vi "Test All.vi"() -> (2 "Failed Tests":i32[](array[numeric]), 3 "All Passed":bool)   [LabVIEW 2017]
uses:
  INI-Static-Variable-Support/LabVIEW-Config/Write Key (Boolean).vi
  INI-Static-Variable-Support/LabVIEW-Config/Read Key (Boolean).vi
  INI-Static-Variable-Support/LabVIEW-Config/Write Key (I32).vi
  INI-Static-Variable-Support/LabVIEW-Config/Read Key (I32).vi
  INI-Static-Variable-Support/LabVIEW-Config/Write Key (U32).vi
  INI-Static-Variable-Support/LabVIEW-Config/Read Key (U32).vi
  INI-Static-Variable-Support/LabVIEW-Config/Write Key (DBL).vi
  INI-Static-Variable-Support/LabVIEW-Config/Read Key (DBL).vi
  INI-Static-Variable-Support/LabVIEW-Config/Write Key (String).vi
  INI-Static-Variable-Support/LabVIEW-Config/Read Key (String).vi
  INI-Static-Variable-Support/LabVIEW-Config/LabVIEW-Config.lvlib
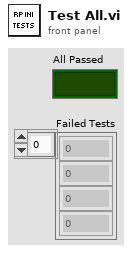
[diagram p1: front panel]
types:
  T1 = typedef "LabVIEW-Config.lvlib/Config.ctl" = cluster{"Path":path, "Lines":string[], "Tokens":enum8{"comment", "section", "key"}[], "Modified?":bool}
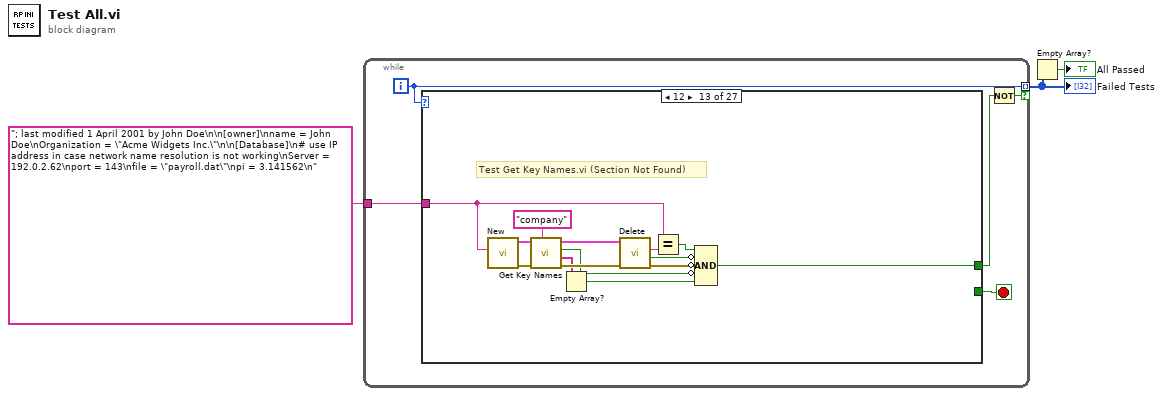
[diagram p0: block diagram]
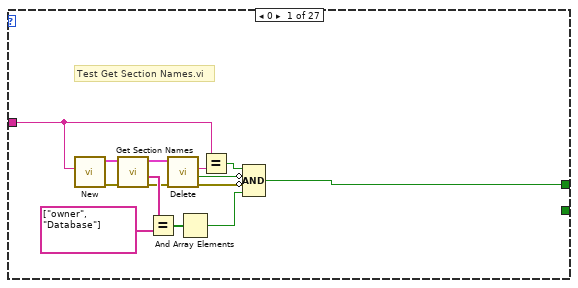
[diagram p2: hidden frame]
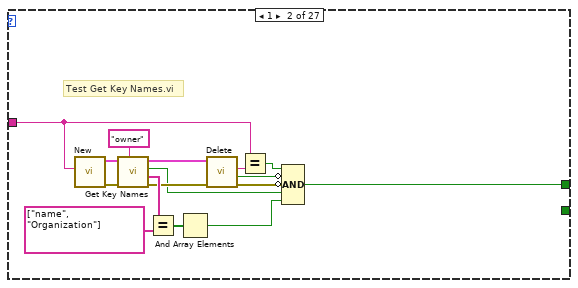
[diagram p3: hidden frame]
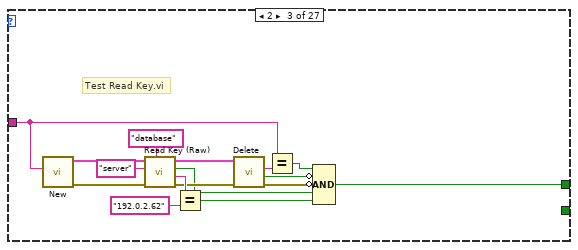
[diagram p4: hidden frame]
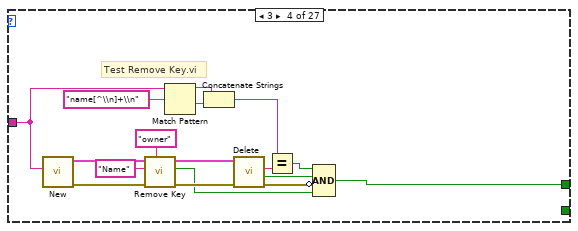
[diagram p5: hidden frame]
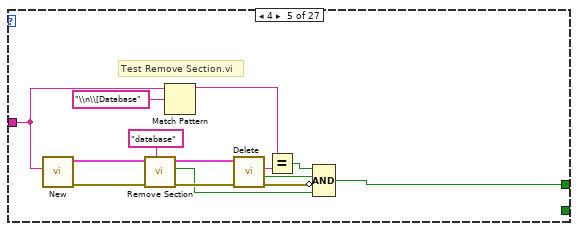
[diagram p6: hidden frame]
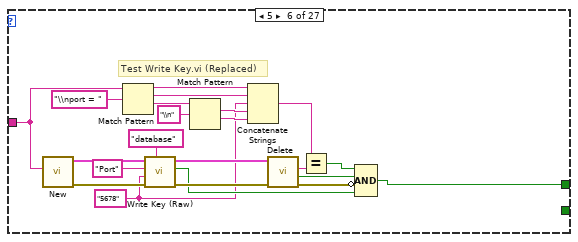
[diagram p7: hidden frame]
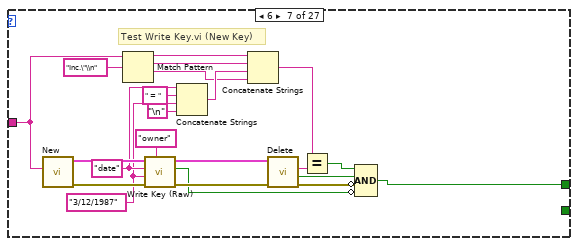
[diagram p8: hidden frame]
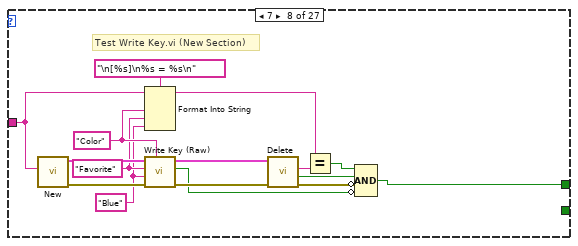
[diagram p9: hidden frame]
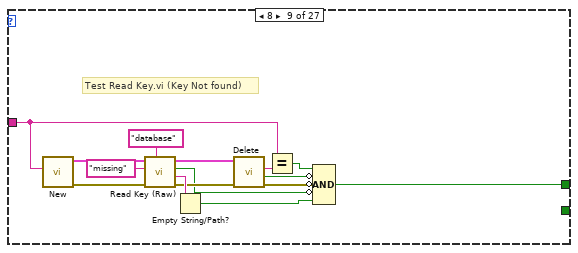
[diagram p10: hidden frame]
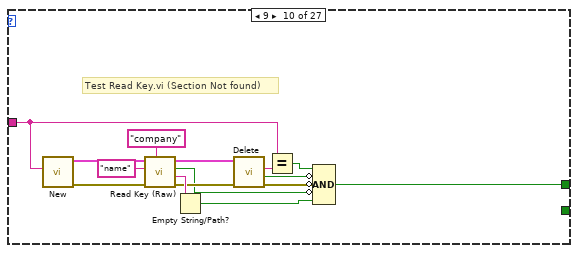
[diagram p11: hidden frame]
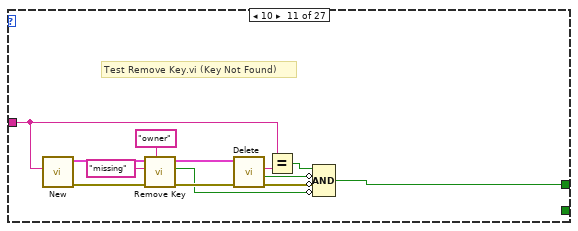
[diagram p12: hidden frame]
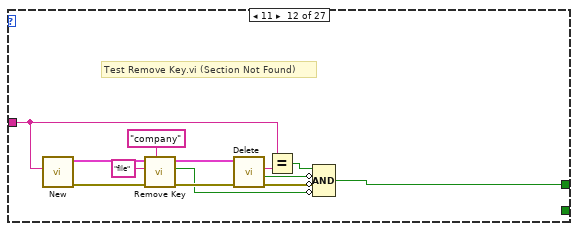
[diagram p13: hidden frame]
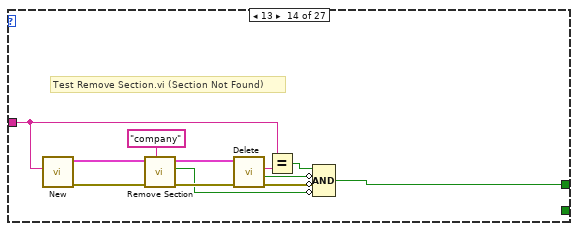
[diagram p14: hidden frame]
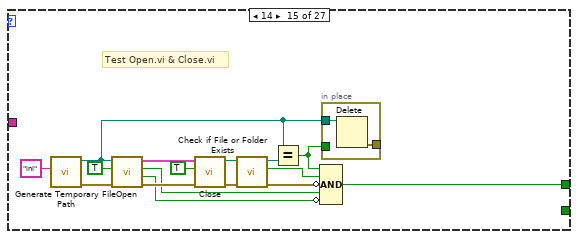
[diagram p15: hidden frame]
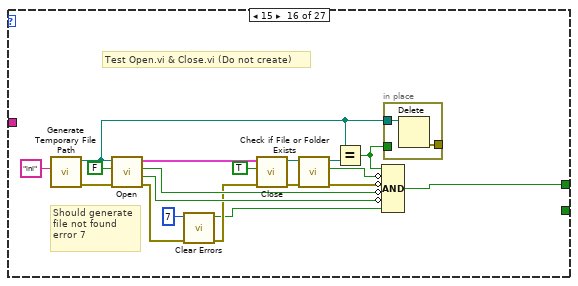
[diagram p16: hidden frame]
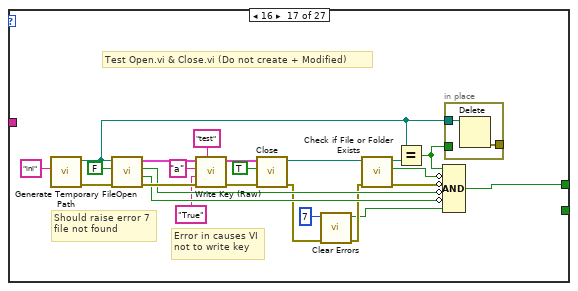
[diagram p17: hidden frame]
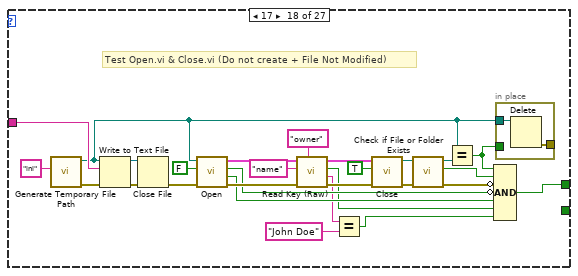
[diagram p18: hidden frame]
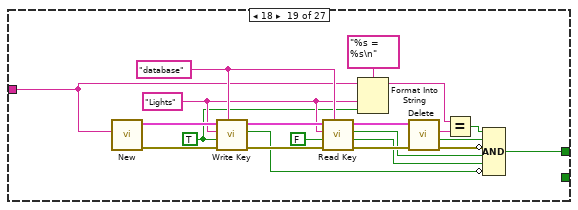
[diagram p19: hidden frame]
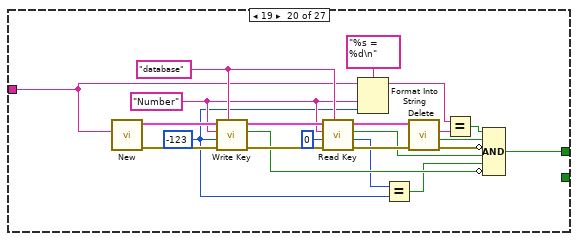
[diagram p20: hidden frame]
diagram:
  n1 = while {
    tunnel: "; last modified 1 April 2001 by John Doe\n\n[owner]\nname = John Doe\nOrganization = \"Acme Widgets Inc.\"\n\n[Database]\n# use IP address in case network name resolution is not working\nServer = 192.0.2.62\nport = 143\nfile = \"payroll.dat\"\npi = 3.141562\n" ("String") -> [w6]
    tunnel: [w7] -> w2 mode=indexing if=w4
    i -> [w7]
    stop <- w8 stop-if-true
    n2 = case shown="12" w7 {
      tunnel: [_ _ _ _ _ _ _ _ _ _ _ _ _ _ _ _ _ _ _ _ _ _ _ _ _ _ TRUE] -> w8
      tunnel: w6 -> [w14 w30 w48 w56 w74 w96 w118 w131 w154 w169 w176 w189 w210 w216 _ _ _ w296 w333 w355 w377 w403 w427 w451 w475 w499 _]
      tunnel: [w10 w24 w43 w62 w76 w98 w120 w137 w149 w164 w179 w192 w205 w218 w234 w255 w283 w313 w325 w348 w370 w396 w420 w444 w468 w492 TRUE] -> w5
      frame 0 {
        # "Test Get Section Names.vi"
        n3 = call "New.vi"("Text"=w14) -> ("error out"=w19:errorcluster, "Config"=w18:T1)  [unwired: 9 in]
        n4 = call "Get Section Names.vi"("error in (no error)"=w19, "Config in"=w18) -> ("error out"=w17:errorcluster, "Section Names"=w22:string[], "Config out"=w16:T1)  [unwired: 7 in]
        n5 = Equal?(x=w22, y=string[] ["owner", "Database"]) -> (x = y?=w20:bool[])
        n6 = call "Delete.vi"("error in (no error)"=w17, "Config"=w16) -> ("error out"=w13:errorcluster, "Modified?"=w9:bool, "Text"=w15:string)  [unwired: 6 in, 1 out]
        n7 = And Array Elements(Boolean array=w20) -> (logical AND=w11:bool)
        n8 = Equal?(x=w14, y=w15) -> (x = y?=w12:bool)
        n9 = Compound Arithmetic op=AND(w12, invert w9, invert w13, w11) -> (w10:bool)
      }
      frame 1 {
        # "Test Get Key Names.vi"
        n10 = call "New.vi"("Text"=w30) -> ("error out"=w35:errorcluster, "Config"=w34:T1)  [unwired: 9 in]
        n11 = call "Get Key Names.vi"("Section Name"="owner", "error in (no error)"=w35, "Config in"=w34) -> ("error out"=w33:errorcluster, "Key Names"=w38:string[], "Section Found?"=w25:bool, "Config out"=w32:T1)  [unwired: 5 in]
        n12 = Equal?(x=w38, y=string[] ["name", "Organization"]) -> (x = y?=w36:bool[])
        n13 = And Array Elements(Boolean array=w36) -> (logical AND=w26:bool)
        n14 = call "Delete.vi"("error in (no error)"=w33, "Config"=w32) -> ("error out"=w28:errorcluster, "Modified?"=w23:bool, "Text"=w31:string)  [unwired: 6 in, 1 out]
        n15 = Equal?(x=w30, y=w31) -> (x = y?=w27:bool)
        n16 = Compound Arithmetic op=AND(w27, invert w23, invert w28, w25, w26) -> (w24:bool)
      }
      frame 2 {
        # "Test Read Key.vi"
        n17 = call "New.vi"("Text"=w48) -> ("error out"=w53:errorcluster, "Config"=w52:T1)  [unwired: 9 in]
        n18 = call "Read Key (Raw).vi"("Section Name"="database", "error in (no error)"=w53, "Key Name"="server", "Config in"=w52) -> ("error out"=w51:errorcluster, "Content"=w54:string, "Key Found?"=w44:bool, "Config out"=w50:T1)  [unwired: 4 in]
        n19 = Equal?(x=w54, y="192.0.2.62") -> (x = y?=w40:bool)
        n20 = call "Delete.vi"("error in (no error)"=w51, "Config"=w50) -> ("error out"=w46:errorcluster, "Modified?"=w39:bool, "Text"=w49:string)  [unwired: 6 in, 1 out]
        n21 = Equal?(x=w48, y=w49) -> (x = y?=w45:bool)
        n22 = Compound Arithmetic op=AND(w45, invert w39, invert w46, w44, w40) -> (w43:bool)
      }
      frame 3 {
        # "Test Remove Key.vi"
        n23 = call "New.vi"("Text"=w56) -> ("error out"=w71:errorcluster, "Config"=w70:T1)  [unwired: 9 in]
        n24 = call "Remove Key.vi"("Section Name"="owner", "error in (no error)"=w71, "Key Name"="Name", "Config in"=w70) -> ("error out"=w69:errorcluster, "Key Found?"=w63:bool, "Config out"=w68:T1)  [unwired: 5 in]
        n25 = Match Pattern(string=w56, regular expression="name[^\\n]+\\n") -> (before substring=w59:string, after substring=w58:string)  [unwired: 1 in, 2 out]
        n26 = Concatenate Strings(w59, w58) -> (w57:string)
        n27 = call "Delete.vi"("error in (no error)"=w69, "Config"=w68) -> ("error out"=w65:errorcluster, "Modified?"=w55:bool, "Text"=w67:string)  [unwired: 6 in, 1 out]
        n28 = Equal?(x=w57, y=w67) -> (x = y?=w64:bool)
        n29 = Compound Arithmetic op=AND(w64, w55, invert w65, w63) -> (w62:bool)
      }
      frame 4 {
        # "Test Remove Section.vi"
        n30 = call "New.vi"("Text"=w74) -> ("error out"=w85:errorcluster, "Config"=w84:T1)  [unwired: 9 in]
        n31 = call "Remove Section.vi"("Section Name"="database", "error in (no error)"=w85, "Config in"=w84) -> ("error out"=w83:errorcluster, "Section Found?"=w77:bool, "Config out"=w82:T1)  [unwired: 6 in]
        n32 = Match Pattern(string=w74, regular expression="\\n\\[Database") -> (before substring=w73:string)  [unwired: 1 in, 3 out]
        n33 = call "Delete.vi"("error in (no error)"=w83, "Config"=w82) -> ("error out"=w79:errorcluster, "Modified?"=w72:bool, "Text"=w81:string)  [unwired: 6 in, 1 out]
        n34 = Equal?(x=w73, y=w81) -> (x = y?=w78:bool)
        n35 = Compound Arithmetic op=AND(w78, w72, invert w79, w77) -> (w76:bool)
      }
      frame 5 {
        w88 = "5678" ("Content")
        # "Test Write Key.vi (Replaced)"
        n36 = call "New.vi"("Text"=w96) -> ("error out"=w107:errorcluster, "Config"=w106:T1)  [unwired: 9 in]
        n37 = Match Pattern(string=w96, regular expression="\\nport = ") -> (before substring=w90:string, match substring=w87:string, after substring=w94:string)  [unwired: 1 in, 1 out]
        n38 = call "Write Key (Raw).vi"("Section Name"="database", "error in (no error)"=w107, "Content"=w88, "Key Name"="Port", "Config in"=w106) -> ("error out"=w105:errorcluster, "Key Replaced?"=w99:bool, "Config out"=w104:T1)  [unwired: 4 in]
        n39 = Match Pattern(string=w94, regular expression="\\n") -> (match substring=w92:string, after substring=w91:string)  [unwired: 1 in, 2 out]
        n40 = Concatenate Strings(w90, w87, w88, w92, w91) -> (w89:string)
        n41 = call "Delete.vi"("error in (no error)"=w105, "Config"=w104) -> ("error out"=w101:errorcluster, "Modified?"=w86:bool, "Text"=w103:string)  [unwired: 6 in, 1 out]
        n42 = Equal?(x=w89, y=w103) -> (x = y?=w100:bool)
        n43 = Compound Arithmetic op=AND(w100, w86, invert w101, w99) -> (w98:bool)
      }
      frame 6 {
        w112 = "3/12/1987" ("Content")
        w114 = "date" ("Key Name")
        # "Test Write Key.vi (New Key)"
        n44 = call "New.vi"("Text"=w118) -> ("error out"=w129:errorcluster, "Config"=w128:T1)  [unwired: 9 in]
        n45 = Match Pattern(string=w118, regular expression="Inc.\"\\n") -> (before substring=w117:string, match substring=w115:string, after substring=w109:string)  [unwired: 1 in, 1 out]
        n46 = call "Write Key (Raw).vi"("Section Name"="owner", "error in (no error)"=w129, "Content"=w112, "Key Name"=w114, "Config in"=w128) -> ("error out"=w127:errorcluster, "Key Replaced?"=w121:bool, "Config out"=w126:T1)  [unwired: 4 in]
        n47 = Concatenate Strings(w114, " = " ("string"), w112, "\n" ("Line Feed Constant")) -> (w111:string)
        n48 = Concatenate Strings(w117, w115, w111, w109) -> (w116:string)
        n49 = call "Delete.vi"("error in (no error)"=w127, "Config"=w126) -> ("error out"=w123:errorcluster, "Modified?"=w108:bool, "Text"=w125:string)  [unwired: 6 in, 1 out]
        n50 = Equal?(x=w116, y=w125) -> (x = y?=w122:bool)
        n51 = Compound Arithmetic op=AND(w122, w108, invert w123, invert w121) -> (w120:bool)
      }
      frame 7 {
        w133 = "Blue" ("Content")
        w134 = "Favorite" ("Key Name")
        w135 = "Color" ("Section Name")
        # "Test Write Key.vi (New Section)"
        n52 = call "New.vi"("Text"=w131) -> ("error out"=w145:errorcluster, "Config"=w144:T1)  [unwired: 9 in]
        n53 = Format Into String(format string="\n[%s]\n%s = %s\n", initial string=w131, w135, w134, w133) -> (resulting string=w130:string)  [unwired: 1 in, 1 out]
        n54 = call "Write Key (Raw).vi"("Section Name"=w135, "error in (no error)"=w145, "Content"=w133, "Key Name"=w134, "Config in"=w144) -> ("error out"=w143:errorcluster, "Key Replaced?"=w138:bool, "Config out"=w142:T1)  [unwired: 4 in]
        n55 = call "Delete.vi"("error in (no error)"=w143, "Config"=w142) -> ("error out"=w140:errorcluster, "Modified?"=w136:bool, "Text"=w141:string)  [unwired: 6 in, 1 out]
        n56 = Equal?(x=w130, y=w141) -> (x = y?=w139:bool)
        n57 = Compound Arithmetic op=AND(w139, w136, invert w140, invert w138) -> (w137:bool)
      }
      frame 8 {
        # "Test Read Key.vi (Key Not found)"
        n58 = call "New.vi"("Text"=w154) -> ("error out"=w159:errorcluster, "Config"=w158:T1)  [unwired: 9 in]
        n59 = call "Read Key (Raw).vi"("Section Name"="database", "error in (no error)"=w159, "Key Name"="missing", "Config in"=w158) -> ("error out"=w157:errorcluster, "Content"=w160:string, "Key Found?"=w150:bool, "Config out"=w156:T1)  [unwired: 4 in]
        n60 = Empty String/Path?(string/path=w160) -> (empty?=w147:bool)
        n61 = call "Delete.vi"("error in (no error)"=w157, "Config"=w156) -> ("error out"=w152:errorcluster, "Modified?"=w146:bool, "Text"=w155:string)  [unwired: 6 in, 1 out]
        n62 = Equal?(x=w154, y=w155) -> (x = y?=w151:bool)
        n63 = Compound Arithmetic op=AND(w151, invert w146, invert w152, invert w150, w147) -> (w149:bool)
      }
      frame 9 {
        # "Test Read Key.vi (Section Not found)"
        n64 = call "New.vi"("Text"=w169) -> ("error out"=w174:errorcluster, "Config"=w173:T1)  [unwired: 9 in]
        n65 = call "Read Key (Raw).vi"("Section Name"="company", "error in (no error)"=w174, "Key Name"="name", "Config in"=w173) -> ("error out"=w172:errorcluster, "Content"=w175:string, "Key Found?"=w165:bool, "Config out"=w171:T1)  [unwired: 4 in]
        n66 = Empty String/Path?(string/path=w175) -> (empty?=w162:bool)
        n67 = call "Delete.vi"("error in (no error)"=w172, "Config"=w171) -> ("error out"=w167:errorcluster, "Modified?"=w161:bool, "Text"=w170:string)  [unwired: 6 in, 1 out]
        n68 = Equal?(x=w169, y=w170) -> (x = y?=w166:bool)
        n69 = Compound Arithmetic op=AND(w166, invert w161, invert w167, invert w165, w162) -> (w164:bool)
      }
      frame 10 {
        # "Test Remove Key.vi (Key Not Found)"
        n70 = call "New.vi"("Text"=w176) -> ("error out"=w188:errorcluster, "Config"=w187:T1)  [unwired: 9 in]
        n71 = call "Remove Key.vi"("Section Name"="owner", "error in (no error)"=w188, "Key Name"="missing", "Config in"=w187) -> ("error out"=w186:errorcluster, "Key Found?"=w180:bool, "Config out"=w185:T1)  [unwired: 5 in]
        n72 = call "Delete.vi"("error in (no error)"=w186, "Config"=w185) -> ("error out"=w182:errorcluster, "Modified?"=w177:bool, "Text"=w184:string)  [unwired: 6 in, 1 out]
        n73 = Equal?(x=w176, y=w184) -> (x = y?=w181:bool)
        n74 = Compound Arithmetic op=AND(w181, invert w177, invert w182, invert w180) -> (w179:bool)
      }
      frame 11 {
        # "Test Remove Key.vi (Section Not Found)"
        n75 = call "New.vi"("Text"=w189) -> ("error out"=w201:errorcluster, "Config"=w200:T1)  [unwired: 9 in]
        n76 = call "Remove Key.vi"("Section Name"="company", "error in (no error)"=w201, "Key Name"="file", "Config in"=w200) -> ("error out"=w199:errorcluster, "Key Found?"=w193:bool, "Config out"=w198:T1)  [unwired: 5 in]
        n77 = call "Delete.vi"("error in (no error)"=w199, "Config"=w198) -> ("error out"=w195:errorcluster, "Modified?"=w190:bool, "Text"=w197:string)  [unwired: 6 in, 1 out]
        n78 = Equal?(x=w189, y=w197) -> (x = y?=w194:bool)
        n79 = Compound Arithmetic op=AND(w194, invert w190, invert w195, invert w193) -> (w192:bool)
      }
      frame 12 {
        # "Test Get Key Names.vi (Section Not Found)"
        n80 = call "New.vi"("Text"=w210) -> ("error out"=w215:errorcluster, "Config"=w214:T1)  [unwired: 9 in]
        n81 = call "Get Key Names.vi"("Section Name"="company", "error in (no error)"=w215, "Config in"=w214) -> ("error out"=w213:errorcluster, "Key Names"=w203:string[], "Section Found?"=w206:bool, "Config out"=w212:T1)  [unwired: 5 in]
        n82 = Empty Array?(array=w203) -> (empty?=w202:bool)
        n83 = call "Delete.vi"("error in (no error)"=w213, "Config"=w212) -> ("error out"=w208:errorcluster, "Modified?"=w204:bool, "Text"=w211:string)  [unwired: 6 in, 1 out]
        n84 = Equal?(x=w210, y=w211) -> (x = y?=w207:bool)
        n85 = Compound Arithmetic op=AND(w207, invert w204, invert w208, invert w206, w202) -> (w205:bool)
      }
      frame 13 {
        # "Test Remove Section.vi (Section Not Found)"
        n86 = call "New.vi"("Text"=w216) -> ("error out"=w227:errorcluster, "Config"=w226:T1)  [unwired: 9 in]
        n87 = call "Remove Section.vi"("Section Name"="company", "error in (no error)"=w227, "Config in"=w226) -> ("error out"=w225:errorcluster, "Section Found?"=w219:bool, "Config out"=w224:T1)  [unwired: 6 in]
        n88 = call "Delete.vi"("error in (no error)"=w225, "Config"=w224) -> ("error out"=w221:errorcluster, "Modified?"=w217:bool, "Text"=w223:string)  [unwired: 6 in, 1 out]
        n89 = Equal?(x=w216, y=w223) -> (x = y?=w220:bool)
        n90 = Compound Arithmetic op=AND(w220, invert w217, invert w221, invert w219) -> (w218:bool)
      }
      frame 14 {
        # "Test Open.vi & Close.vi"
        n91 = call <vilib>:"Generate Temporary File Path.vi"("Temporary File Extension (tmp)"="ini") -> ("error out"=w240:errorcluster, "Unique Temporary File Path"=w233:path)  [unwired: 9 in]
        n92 = call "Open.vi"("error in (no error)"=w240, "Create if not exists? (T)"=TRUE, "Path"=w233) -> ("error out"=w243:errorcluster, "File Exists?"=w235:bool, "File Created?"=w236:bool, "Config"=w242:T1)  [unwired: 5 in]
        n93 = call "Close.vi"("error in (no error)"=w243, "Write if modified? (T)"=TRUE, "Config"=w242) -> ("error out"=w237:errorcluster, "Path"=w230:path)  [unwired: 7 in]
        n94 = call <vilib>:"Check if File or Folder Exists.vi"("error in (no error)"=w237, "path"=w230) -> ("error out"=w231:errorcluster, "file or folder exists?"=w228:bool, "dup path"=w229:path)  [unwired: 7 in]
        n95 = Equal?(x=w233, y=w229) -> (x = y?=w232:bool)
        n96 = Compound Arithmetic op=AND(w232, w228, invert w231, w236, invert w235) -> (w234:bool)
        n97 = in-place {
          in-place-border: w233 -> [w245]
          in-place-border: w232 -> [_]
          in-place-border: [w244] -> _
          n98 = Delete(path (use dialog)=w245) -> (error out=w244:errorcluster)  [unwired: 4 in, 2 out]
        }
      }
      frame 15 {
        # "Should generate\nfile not found\nerror 7"
        # "Test Open.vi & Close.vi (Do not create)"
        n99 = call <vilib>:"Generate Temporary File Path.vi"("Temporary File Extension (tmp)"="ini") -> ("error out"=w261:errorcluster, "Unique Temporary File Path"=w254:path)  [unwired: 9 in]
        n100 = call "Open.vi"("error in (no error)"=w261, "Create if not exists? (T)"=FALSE, "Path"=w254) -> ("error out"=w264:errorcluster, "File Exists?"=w256:bool, "File Created?"=w257:bool, "Config"=w263:T1)  [unwired: 5 in]
        n101 = call <vilib>:"Clear Errors.vi"("error in (no error)"=w264, "specific error code to clear (0: all)"=7) -> ("error out"=w248:errorcluster, "specific error cleared?"=w246:bool)  [unwired: 4 in]
        n102 = call "Close.vi"("error in (no error)"=w248, "Write if modified? (T)"=TRUE, "Config"=w263) -> ("error out"=w258:errorcluster, "Path"=w251:path)  [unwired: 7 in]
        n103 = call <vilib>:"Check if File or Folder Exists.vi"("error in (no error)"=w258, "path"=w251) -> ("error out"=w252:errorcluster, "file or folder exists?"=w249:bool, "dup path"=w250:path)  [unwired: 7 in]
        n104 = Equal?(x=w254, y=w250) -> (x = y?=w253:bool)
        n105 = Compound Arithmetic op=AND(w253, invert w249, invert w252, invert w257, invert w256, w246) -> (w255:bool)
        n106 = in-place {
          in-place-border: w254 -> [w266]
          in-place-border: w253 -> [_]
          in-place-border: [w265] -> _
          n107 = Delete(path (use dialog)=w266) -> (error out=w265:errorcluster)  [unwired: 4 in, 2 out]
        }
      }
      frame 16 {
        # "Error in causes VI\nnot to write key"
        # "Should raise error 7\nfile not found"
        # "Test Open.vi & Close.vi (Do not create + Modified)"
        n108 = call <vilib>:"Generate Temporary File Path.vi"("Temporary File Extension (tmp)"="ini") -> ("error out"=w288:errorcluster, "Unique Temporary File Path"=w282:path)  [unwired: 9 in]
        n109 = call "Open.vi"("error in (no error)"=w288, "Create if not exists? (T)"=FALSE, "Path"=w282) -> ("error out"=w290:errorcluster, "File Exists?"=w284:bool, "File Created?"=w285:bool, "Config"=w275:T1)  [unwired: 5 in]
        n110 = call "Write Key (Raw).vi"("Section Name"="test", "error in (no error)"=w290, "Content"="True", "Key Name"="a", "Config in"=w275) -> ("error out"=w276:errorcluster, "Config out"=w274:T1)  [unwired: 4 in, 1 out]
        n111 = call "Close.vi"("error in (no error)"=w276, "Write if modified? (T)"=TRUE, "Config"=w274) -> ("error out"=w269:errorcluster, "Path"=w279:path)  [unwired: 7 in]
        n112 = call <vilib>:"Clear Errors.vi"("error in (no error)"=w269, "specific error code to clear (0: all)"=7) -> ("error out"=w268:errorcluster, "specific error cleared?"=w267:bool)  [unwired: 4 in]
        n113 = call <vilib>:"Check if File or Folder Exists.vi"("error in (no error)"=w268, "path"=w279) -> ("error out"=w280:errorcluster, "file or folder exists?"=w277:bool, "dup path"=w278:path)  [unwired: 7 in]
        n114 = Equal?(x=w282, y=w278) -> (x = y?=w281:bool)
        n115 = Compound Arithmetic op=AND(w281, invert w277, invert w280, invert w285, invert w284, w267) -> (w283:bool)
        n116 = in-place {
          in-place-border: w282 -> [w292]
          in-place-border: w281 -> [_]
          in-place-border: [w291] -> _
          n117 = Delete(path (use dialog)=w292) -> (error out=w291:errorcluster)  [unwired: 4 in, 2 out]
        }
      }
      frame 17 {
        # "Test Open.vi & Close.vi (Do not create + File Not Modified)"
        n118 = call <vilib>:"Generate Temporary File Path.vi"("Temporary File Extension (tmp)"="ini") -> ("error out"=w318:errorcluster, "Unique Temporary File Path"=w293:path)  [unwired: 9 in]
        n119 = Write to Text File(file (use dialog)=w293, text=w296, error in=w318) -> (refnum out=w294:refnum<file>, error out=w297:errorcluster)  [unwired: 1 in, 1 out]
        n120 = Close File(refnum=w294, error in=w297) -> (error out=w295:errorcluster)  [unwired: 1 out]
        n121 = call "Open.vi"("error in (no error)"=w295, "Create if not exists? (T)"=FALSE, "Path"=w293) -> ("error out"=w320:errorcluster, "File Exists?"=w314:bool, "File Created?"=w315:bool, "Config"=w306:T1)  [unwired: 5 in]
        n122 = call "Read Key (Raw).vi"("Section Name"="owner", "error in (no error)"=w320, "Key Name"="name", "Config in"=w306) -> ("error out"=w307:errorcluster, "Content"=w300:string, "Key Found?"=w301:bool, "Config out"=w305:T1)  [unwired: 4 in]
        n123 = Equal?(x=w300, y="John Doe") -> (x = y?=w298:bool)
        n124 = call "Close.vi"("error in (no error)"=w307, "Write if modified? (T)"=TRUE, "Config"=w305) -> ("error out"=w302:errorcluster, "Path"=w310:path)  [unwired: 7 in]
        n125 = call <vilib>:"Check if File or Folder Exists.vi"("error in (no error)"=w302, "path"=w310) -> ("error out"=w311:errorcluster, "file or folder exists?"=w308:bool, "dup path"=w309:path)  [unwired: 7 in]
        n126 = Equal?(x=w293, y=w309) -> (x = y?=w312:bool)
        n127 = Compound Arithmetic op=AND(w312, w308, invert w311, invert w315, w314, w301, w298) -> (w313:bool)
        n128 = in-place {
          in-place-border: w293 -> [w322]
          in-place-border: w312 -> [_]
          in-place-border: [w321] -> _
          n129 = Delete(path (use dialog)=w322) -> (error out=w321:errorcluster)  [unwired: 4 in, 2 out]
        }
      }
      frame 18 {
        w323 = TRUE ("Value")
        w332 = "Lights" ("Key Name")
        w337 = "database" ("Section Name")
        n130 = call "New.vi"("Text"=w333) -> ("error out"=w343:errorcluster, "Config"=w339:T1)  [unwired: 9 in]
        n131 = call-poly "Write Key.vi"("Section Name"=w337, "error in (no error)"=w343, "Value"=w323, "Key Name"=w332, "Config in"=w339) -> ("error out"=w340:errorcluster, "Key Replaced?"=w326:bool, "Config out"=w338:T1)  [unwired: 4 in]
        n132 = call-poly "Read Key.vi"("Section Name"=w337, "error in (no error)"=w340, "Default"=FALSE, "Key Name"=w332, "Config in"=w338) -> ("error out"=w342:errorcluster, "Value"=w327:bool, "Key Found?"=w328:bool, "Config out"=w341:T1)  [unwired: 3 in]
        n133 = Format Into String(format string="%s = %s\n", initial string=w333, w332, w323) -> (resulting string=w330:string)  [unwired: 1 in, 1 out]
        n134 = call "Delete.vi"("error in (no error)"=w342, "Config"=w341) -> ("error out"=w336:errorcluster, "Modified?"=w335:bool, "Text"=w334:string)  [unwired: 6 in, 1 out]
        n135 = Equal?(x=w330, y=w334) -> (x = y?=w329:bool)
        n136 = Compound Arithmetic op=AND(w329, w335, invert w336, w328, w327, invert w326) -> (w325:bool)
      }
      frame 19 {
        w346 = -123 ("Value")
        w354 = "Number" ("Key Name")
        w359 = "database" ("Section Name")
        n137 = call "New.vi"("Text"=w355) -> ("error out"=w365:errorcluster, "Config"=w361:T1)  [unwired: 9 in]
        n138 = call-poly "Write Key.vi"("Section Name"=w359, "error in (no error)"=w365, "Value"=w346, "Key Name"=w354, "Config in"=w361) -> ("error out"=w362:errorcluster, "Key Replaced?"=w349:bool, "Config out"=w360:T1)  [unwired: 4 in]
        n139 = call-poly "Read Key.vi"("Section Name"=w359, "error in (no error)"=w362, "Default"=0, "Key Name"=w354, "Config in"=w360) -> ("error out"=w364:errorcluster, "Value"=w345:i32, "Key Found?"=w350:bool, "Config out"=w363:T1)  [unwired: 3 in]
        n140 = Format Into String(format string="%s = %d\n", initial string=w355, w354, w346) -> (resulting string=w352:string)  [unwired: 1 in, 1 out]
        n141 = Equal?(x=w345, y=w346) -> (x = y?=w344:bool)
        n142 = call "Delete.vi"("error in (no error)"=w364, "Config"=w363) -> ("error out"=w358:errorcluster, "Modified?"=w357:bool, "Text"=w356:string)  [unwired: 6 in, 1 out]
        n143 = Equal?(x=w352, y=w356) -> (x = y?=w351:bool)
        n144 = Compound Arithmetic op=AND(w351, w357, invert w358, w350, w344, invert w349) -> (w348:bool)
      }
      frame 20 {
        w369 = u32 5 ("Value")
        w376 = "Number" ("Key Name")
        w381 = "database" ("Section Name")
        n145 = call "New.vi"("Text"=w377) -> ("error out"=w387:errorcluster, "Config"=w383:T1)  [unwired: 9 in]
        n146 = call-poly "Write Key.vi"("Section Name"=w381, "error in (no error)"=w387, "Value"=w369, "Key Name"=w376, "Config in"=w383) -> ("error out"=w384:errorcluster, "Key Replaced?"=w371:bool, "Config out"=w382:T1)  [unwired: 4 in]
        n147 = call-poly "Read Key.vi"("Section Name"=w381, "error in (no error)"=w384, "Default"=u32 0, "Key Name"=w376, "Config in"=w382) -> ("error out"=w386:errorcluster, "Value"=w368:u32, "Key Found?"=w372:bool, "Config out"=w385:T1)  [unwired: 3 in]
        n148 = Format Into String(format string="%s = %d\n", initial string=w377, w376, w369) -> (resulting string=w374:string)  [unwired: 1 in, 1 out]
        n149 = Equal?(x=w368, y=w369) -> (x = y?=w367:bool)
        n150 = call "Delete.vi"("error in (no error)"=w386, "Config"=w385) -> ("error out"=w380:errorcluster, "Modified?"=w379:bool, "Text"=w378:string)  [unwired: 6 in, 1 out]
        n151 = Equal?(x=w374, y=w378) -> (x = y?=w373:bool)
        n152 = Compound Arithmetic op=AND(w373, w379, invert w380, w372, w367, invert w371) -> (w370:bool)
      }
      frame 21 {
        w395 = 3.1415 ("Value")
        w402 = "Number" ("Key Name")
        w407 = "database" ("Section Name")
        n153 = call "New.vi"("Text"=w403) -> ("error out"=w413:errorcluster, "Config"=w409:T1)  [unwired: 9 in]
        n154 = call-poly "Write Key.vi"("Format String ('%#.12g')"="%.4f", "Section Name"=w407, "error in (no error)"=w413, "Value"=w395, "Key Name"=w402, "Config in"=w409) -> ("error out"=w410:errorcluster, "Key Replaced?"=w397:bool, "Config out"=w408:T1)  [unwired: 3 in]
        n155 = call-poly "Read Key.vi"("Section Name"=w407, "error in (no error)"=w410, "Default"=0.0, "Key Name"=w402, "Config in"=w408) -> ("error out"=w412:errorcluster, "Value"=w394:dbl, "Key Found?"=w398:bool, "Config out"=w411:T1)  [unwired: 3 in]
        n156 = Format Into String(format string="%s = %.4f\n", initial string=w403, w402, w395) -> (resulting string=w400:string)  [unwired: 1 in, 1 out]
        n157 = Subtract(x=w394, y=w395) -> (x-y=w392:dbl)
        n158 = call "Delete.vi"("error in (no error)"=w412, "Config"=w411) -> ("error out"=w406:errorcluster, "Modified?"=w405:bool, "Text"=w404:string)  [unwired: 6 in, 1 out]
        n159 = In Range and Coerce(upper limit=0.0001, x=w392, lower limit=-0.0001 ("upper limit")) -> (In Range?=w391:bool)  [unwired: 1 out]
        n160 = Equal?(x=w400, y=w404) -> (x = y?=w399:bool)
        n161 = Compound Arithmetic op=AND(w399, w405, invert w406, w398, w391, invert w397) -> (w396:bool)
      }
      frame 22 {
        w418 = "a b2"
        w426 = "String" ("Key Name")
        w431 = "database" ("Section Name")
        n162 = call "New.vi"("Text"=w427) -> ("error out"=w437:errorcluster, "Config"=w433:T1)  [unwired: 9 in]
        n163 = call-poly "Write Key.vi"("Write Raw String? (F)"=FALSE, "Section Name"=w431, "error in (no error)"=w437, "Value"=w418, "Key Name"=w426, "Config in"=w433) -> ("error out"=w434:errorcluster, "Key Replaced?"=w421:bool, "Config out"=w432:T1)  [unwired: 3 in]
        n164 = call-poly "Read Key.vi"("Read Raw String? (F)"=FALSE, "Section Name"=w431, "error in (no error)"=w434, "Default"="", "Key Name"=w426, "Config in"=w432) -> ("error out"=w436:errorcluster, "Value"=w419:string, "Key Found?"=w422:bool, "Config out"=w435:T1)  [unwired: 2 in]
        n165 = Format Into String(format string="%s = \"%s\"\n", initial string=w427, w426, w418) -> (resulting string=w424:string)  [unwired: 1 in, 1 out]
        n166 = Equal?(x=w419, y=w418) -> (x = y?=w417:bool)
        n167 = call "Delete.vi"("error in (no error)"=w436, "Config"=w435) -> ("error out"=w430:errorcluster, "Modified?"=w429:bool, "Text"=w428:string)  [unwired: 6 in, 1 out]
        n168 = Equal?(x=w424, y=w428) -> (x = y?=w423:bool)
        n169 = Compound Arithmetic op=AND(w423, w429, invert w430, w422, w417, invert w421) -> (w420:bool)
      }
      frame 23 {
        w442 = "C:\\b2"
        w450 = "String" ("Key Name")
        w455 = "database" ("Section Name")
        n170 = call "New.vi"("Text"=w451) -> ("error out"=w461:errorcluster, "Config"=w457:T1)  [unwired: 9 in]
        n171 = call-poly "Write Key.vi"("Write Raw String? (F)"=TRUE, "Section Name"=w455, "error in (no error)"=w461, "Value"=w442, "Key Name"=w450, "Config in"=w457) -> ("error out"=w458:errorcluster, "Key Replaced?"=w445:bool, "Config out"=w456:T1)  [unwired: 3 in]
        n172 = call-poly "Read Key.vi"("Read Raw String? (F)"=TRUE, "Section Name"=w455, "error in (no error)"=w458, "Default"="", "Key Name"=w450, "Config in"=w456) -> ("error out"=w460:errorcluster, "Value"=w443:string, "Key Found?"=w446:bool, "Config out"=w459:T1)  [unwired: 2 in]
        n173 = Format Into String(format string="%s = \"%s\"\n", initial string=w451, w450, w442) -> (resulting string=w448:string)  [unwired: 1 in, 1 out]
        n174 = Equal?(x=w443, y=w442) -> (x = y?=w441:bool)
        n175 = call "Delete.vi"("error in (no error)"=w460, "Config"=w459) -> ("error out"=w454:errorcluster, "Modified?"=w453:bool, "Text"=w452:string)  [unwired: 6 in, 1 out]
        n176 = Equal?(x=w448, y=w452) -> (x = y?=w447:bool)
        n177 = Compound Arithmetic op=AND(w447, w453, invert w454, w446, w441, invert w445) -> (w444:bool)
      }
      frame 24 {
        w466 = "C:\\b2"
        w474 = "String" ("Key Name")
        w479 = "database" ("Section Name")
        n178 = call "New.vi"("Text"=w475) -> ("error out"=w485:errorcluster, "Config"=w481:T1)  [unwired: 9 in]
        n179 = call-poly "Write Key.vi"("Write Raw String? (F)"=FALSE, "Section Name"=w479, "error in (no error)"=w485, "Value"=w466, "Key Name"=w474, "Config in"=w481) -> ("error out"=w482:errorcluster, "Key Replaced?"=w469:bool, "Config out"=w480:T1)  [unwired: 3 in]
        n180 = call-poly "Read Key.vi"("Read Raw String? (F)"=FALSE, "Section Name"=w479, "error in (no error)"=w482, "Default"="", "Key Name"=w474, "Config in"=w480) -> ("error out"=w484:errorcluster, "Value"=w467:string, "Key Found?"=w470:bool, "Config out"=w483:T1)  [unwired: 2 in]
        n181 = Format Into String(format string="%s = \"C:\\\\\\\\b2\"\n", initial string=w475, w474) -> (resulting string=w472:string)  [unwired: 1 in, 1 out]
        n182 = Equal?(x=w467, y=w466) -> (x = y?=w465:bool)
        n183 = call "Delete.vi"("error in (no error)"=w484, "Config"=w483) -> ("error out"=w478:errorcluster, "Modified?"=w477:bool, "Text"=w476:string)  [unwired: 6 in, 1 out]
        n184 = Equal?(x=w472, y=w476) -> (x = y?=w471:bool)
        n185 = Compound Arithmetic op=AND(w471, w477, invert w478, w470, w465, invert w469) -> (w468:bool)
      }
      frame 25 {
        w486 = "C:\\b2"
        w498 = "String" ("Key Name")
        w503 = "database" ("Section Name")
        n186 = call "New.vi"("Text"=w499) -> ("error out"=w509:errorcluster, "Config"=w505:T1)  [unwired: 9 in]
        n187 = call-poly "Write Key.vi"("Write Raw String? (F)"=TRUE, "Section Name"=w503, "error in (no error)"=w509, "Value"=w486, "Key Name"=w498, "Config in"=w505) -> ("error out"=w506:errorcluster, "Key Replaced?"=w493:bool, "Config out"=w504:T1)  [unwired: 3 in]
        n188 = call-poly "Read Key.vi"("Read Raw String? (F)"=FALSE, "Section Name"=w503, "error in (no error)"=w506, "Default"="", "Key Name"=w498, "Config in"=w504) -> ("error out"=w508:errorcluster, "Value"=w491:string, "Key Found?"=w494:bool, "Config out"=w507:T1)  [unwired: 2 in]
        n189 = Format Into String(format string="%s = \"%s\"\n", initial string=w499, w498, w486) -> (resulting string=w496:string)  [unwired: 1 in, 1 out]
        n190 = Equal?(x=w491, y=w486) -> (x = y?=w490:bool)
        n191 = call "Delete.vi"("error in (no error)"=w508, "Config"=w507) -> ("error out"=w502:errorcluster, "Modified?"=w501:bool, "Text"=w500:string)  [unwired: 6 in, 1 out]
        n192 = Equal?(x=w496, y=w500) -> (x = y?=w495:bool)
        n193 = Compound Arithmetic op=AND(w495, w501, invert w502, w494, w490, invert w493) -> (w492:bool)
      }
      frame Default {
      }
    }
    n194 = Not(x=w5) -> (.not. x?=w4:bool)
  }
  "Failed Tests" <- w2
  n195 = Empty Array?(array=w2) -> (empty?=→"All Passed":bool)
